vi "WinCI Initialize.vi"(8 "error in (no error)":errorcluster, 11 "provider name":string) -> (0 "error out":errorcluster, 2 "suppCaps":u32)   [LabVIEW 2020, in "NI_SCC_WinCI.lvlib"]
uses:
  <vilib>/SourceControl/Providers/WinCI/NI_SCC_WinCI.lvlib
  <vilib>/SourceControl/support/SCCSup Message Strings GLBL.vi
panel:
  out "active connection?":bool
  out "providerFound":i32
  out "lErr":i32
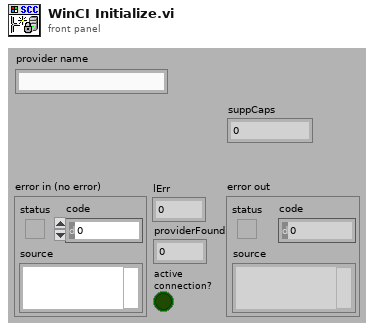
[diagram p1: front panel]
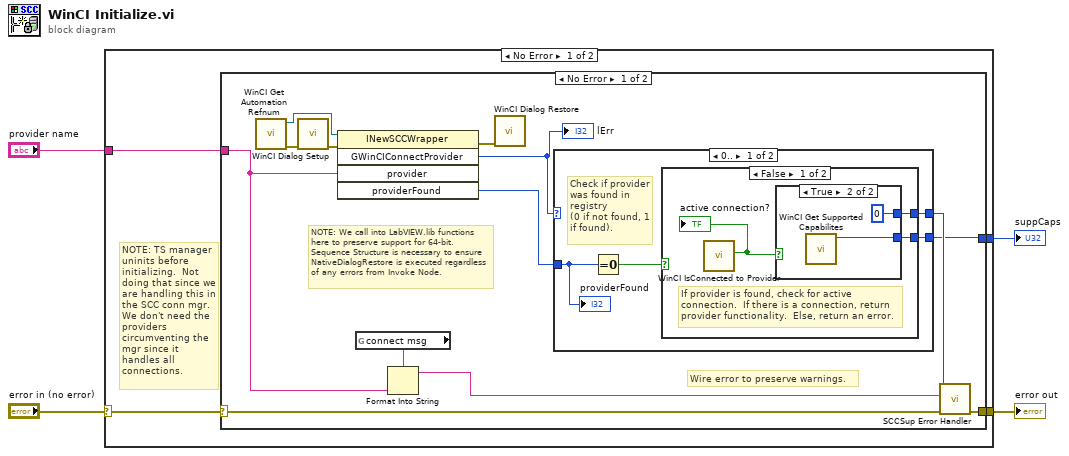
[diagram p0: block diagram]
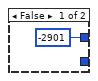
[diagram p2: hidden frame]
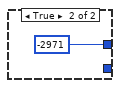
[diagram p3: hidden frame]
diagram:
  n1 = case shown="No Error" "error in (no error)" {
    selector: "error in (no error)" -> [w6 w35]
    tunnel: [w7 w35] -> w2
    tunnel: "provider name" -> [w8 _]
    tunnel: [w5 _] -> w1
    frame No Error {
      # "NOTE: TS manager uninits before initializing.  Not doing that since we are handling this in the SCC conn mgr.  We don't need the providers circumventing the mgr since it handles all connections."
      n2 = case shown="No Error" w6 {
        selector: w6 -> [w17 w34]
        tunnel: w8 -> [w15 _]
        tunnel: [w21 w34] -> w7
        tunnel: [w16 _] -> w5
        frame No Error {
          # "NOTE: We call into LabVIEW.lib functions here to preserve support for 64-bit. Sequence Structure is necessary to ensure NativeDialogRestore is executed regardless of any errors from Invoke Node."
          # "Wire error to preserve warnings."
          n3 = call <vilib>:"WinCI Get Automation Refnum.vi"() -> ("error out"=w11:errorcluster, "automation refnum"=w12:refnum<k7>)  [unwired: 10 out]
          n4 = call <vilib>:"WinCI Dialog Setup.vi"("error in"=w11) -> ("error out"=w10:errorcluster)  [unwired: 10 out]
          n5 = invoke class="INewSCCWrapper" method="GWinCIConnectProvider"(reference=w12, error in=w10, "provider"=w15) -> (error out=w9:errorcluster, "GWinCIConnectProvider"=w14:i32, "providerFound"=w13:i32)  [unwired: 2 in, 2 out]
          "lErr" <- w14
          n6 = global read "SCCSup Message Strings GLBL.vi" "connect msg"() -> (w19:string)
          n7 = Format Into String(format string=w19, w15) -> (resulting string=w18:string)  [unwired: 2 in, 1 out]
          n8 = call <vilib>:"WinCI Dialog Restore.vi"("error in"=w9) -> ()  [unwired: 11 out]
          n9 = case shown="0.." w14 {
            selector: w14 -> [_ w33]
            tunnel: w13 -> [w23 _]
            tunnel: [w24 w33] -> w20
            tunnel: [w22 _] -> w16
            frame 0.. {
              # "Check if provider was found in registry\n(0 if not found, 1 if found)."
              n10 = Equal To 0?(x=w23) -> (x = 0?=w25:bool)
              n11 = case shown="False" w25 {
                tunnel: [w28 -2971 ("t")] -> w24
                tunnel: [w27 _] -> w22
                frame False {
                  # "If provider is found, check for active connection.  If there is a connection, return provider functionality.  Else, return an error."
                  n12 = call <vilib>:"WinCI IsConnected to Provider.vi"() -> ("active connection?"=w26:bool)  [unwired: 1 in, 10 out]
                  "active connection?" <- w26
                  n13 = case shown="True" w26 {
                    tunnel: [_ w30] -> w27
                    tunnel: [-2901 ("t") 0 ("t")] -> w28
                    frame False {
                    }
                    frame True {
                      n14 = call <vilib>:"WinCI Get Supported Capabilites.vi"() -> ("suppCaps"=w30:u32)  [unwired: 1 in, 10 out]
                    }
                  }
                }
                frame True {
                }
              }
              "providerFound" <- w23
            }
            frame Default {
              # "Error occured in wrapper."
            }
          }
          n15 = call <vilib>:"SCCSup Error Handler.vi"("error in (no error)"=w17, "operation message"=w18, "scc error code"=w20) -> ("error out"=w21:errorcluster)  [unwired: 1 in, 7 out]
        }
        frame Error {
        }
      }
    }
    frame Error {
    }
  }
  "error out" <- w2
  "suppCaps" <- w1
